vi "REWORK_parse_rework_commit_response.vi"(8 "error_in":errorcluster, 11 "sql_results_in":variant) -> (0 "error_out":errorcluster)   [LabVIEW 2019]
uses:
  _misc/AULocalize/SubVIs/Get Localized Phrase Compact Interface 0D.vi
  <vilib>/addons/database/_DB Variant To Data/Database Variant To Data.xnode
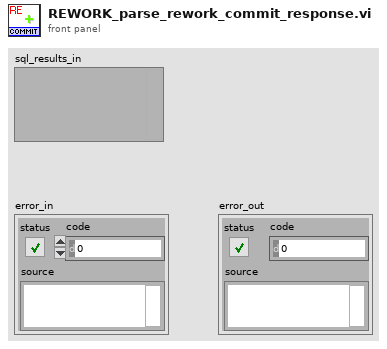
[diagram p1: front panel]
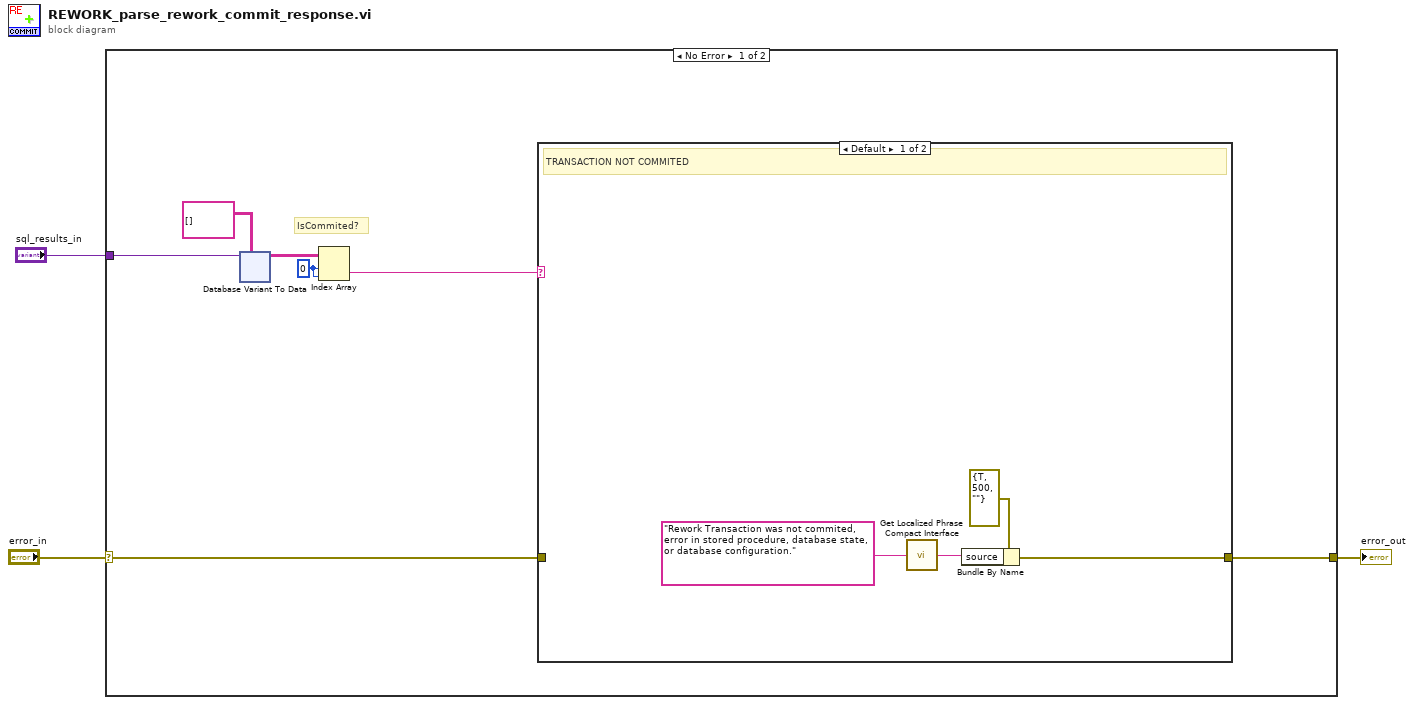
[diagram p0: block diagram]
diagram:
  n1 = case shown="No Error" "error_in" {
    selector: "error_in" -> [w8 w48]
    tunnel: "sql_results_in" -> [w4 _]
    tunnel: [w7 w48] -> w2
    frame No Error {
      w6 = 0 ("index (row)")
      # "IsCommited?"
      n2 = xnode "Database Variant To Data"("database variant"=w4, "type"=string[][] []) -> ("data"=w9:string[][])  [unwired: 1 in, 1 out]
      n3 = Index Array(array=w9, index (row)=w6, index (col)=w6) -> (element=w5:string)
      n4 = case shown="Default" w5 {
        tunnel: w8 -> [_ w47]
        tunnel: [w45 w47] -> w7
        frame Default {
          # "TRANSACTION NOT COMMITED"
          n5 = call-poly "Get Localized Phrase Compact Interface.vi"("Key"="Rework Transaction was not commited, error in stored procedure, database state, or database configuration." ("source")) -> ("Translated Phrase"=w44:string)
          n6 = Bundle By Name(cluster=errorcluster {"status"=TRUE, "code"=500, "source"=""} ("error IO"), "source"=w44) -> (w45:errorcluster)
        }
        frame "1" {
          # "TRANSACTION COMMITED"
        }
      }
    }
    frame Error {
    }
  }
  "error_out" <- w2
